vi "Obtain Request Events.vi"(8 "error in":errorcluster, 10 "Create New? (F)":bool) -> (0 "error out":errorcluster, 2 "USB IO Request Events":T1)   [LabVIEW 2025, in "USB IO.lvlib"]
doc: "This VI Obtains/Creates the Requests events that will be used for other modules to communicate with the module that owns this VI. These Requests events will be accessed only via Public API methods for this module.\n\n<b>NOTE</b>: The contents of this VI are automatically generated and modified by the <b>Tools > DQMH Consortium > DQMH</b> utilities. Consider using those utilities instead of making your own modifications to this VI.\n_____\nBased on DQMH Dev Tools: Project Template 7.1.2.1547."
uses:
  USB IO.lvlib
  Request Events--cluster.ctl
  Stop Argument--cluster.ctl
  Show Panel Argument--cluster.ctl
  Hide Panel Argument--cluster.ctl
  Show Diagram Argument--cluster.ctl
  Get Module Execution Status Argument--cluster.ctl
  Display Lines Argument--cluster.ctl
  Display Lines (Reply Payload)--cluster.ctl
  select child Argument--cluster.ctl
  Classes/Hardware Selection.ctl
  select child (Reply Payload)--cluster.ctl
  read config Argument--cluster.ctl
  read config (Reply Payload)--cluster.ctl
  init Argument--cluster.ctl
  init (Reply Payload)--cluster.ctl
  init device Argument--cluster.ctl
  init device (Reply Payload)--cluster.ctl
  stop device Argument--cluster.ctl
  stop device (Reply Payload)--cluster.ctl
  analog read Argument--cluster.ctl
  analog read (Reply Payload)--cluster.ctl
  Controls/Numeric Voltage.ctl
  digital write Argument--cluster.ctl
  digital write (Reply Payload)--cluster.ctl
panel:
  # "NOTE: The contents of this VI are automatically generated and modified by the Tools > DQMH Consortium > DQMH utilities. Consider using those utilities instead of making your own modifications to this VI."
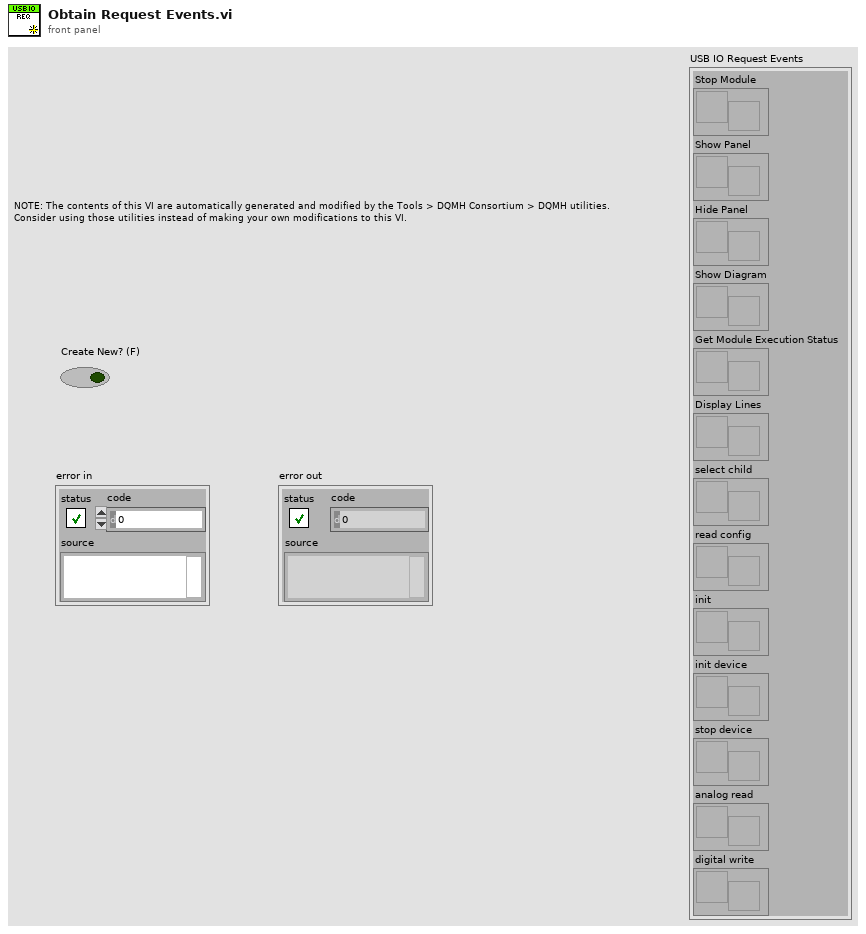
[diagram p1: front panel]
types:
  T1 = typedef "USB IO.lvlib/Request Events--cluster.ctl" = cluster{"Stop Module":refnum<user-event>, "Show Panel":refnum<user-event>, "Hide Panel":refnum<user-event>, "Show Diagram":refnum<user-event>, "Get Module Execution Status":refnum<user-event>, "Display Lines":refnum<user-event>, "select child":refnum<user-event>, "read config":refnum<user-event>, "init":refnum<user-event>, "init device":refnum<user-event>, "stop device":refnum<user-event>, "analog read":refnum<user-event>, "digital write":refnum<user-event>}
  T2 = typedef "USB IO.lvlib/digital write Argument--cluster.ctl" = cluster{"Module ID":i32, "Line":string, "On/Off":bool, "Wait Notifier":refnum<notifier>, "wait for reply":bool}
  T3 = typedef "USB IO.lvlib/analog read Argument--cluster.ctl" = cluster{"Module ID":i32, "Line":string, "Wait Notifier":refnum<notifier>, "wait for reply":bool}
  T4 = typedef "USB IO.lvlib/stop device Argument--cluster.ctl" = cluster{"Module ID":i32, "Wait Notifier":refnum<notifier>, "wait for reply":bool}
  T5 = typedef "USB IO.lvlib/init device Argument--cluster.ctl" = cluster{"Module ID":i32, "Variant":variant, "Wait Notifier":refnum<notifier>, "wait for reply":bool}
  T6 = typedef "USB IO.lvlib/init Argument--cluster.ctl" = cluster{"Module ID":i32, "Wait Notifier":refnum<notifier>, "wait for reply":bool}
  T7 = typedef "USB IO.lvlib/read config Argument--cluster.ctl" = cluster{"Module ID":i32, "Path":path, "Wait Notifier":refnum<notifier>, "wait for reply":bool}
  T8 = typedef "USB IO.lvlib/select child Argument--cluster.ctl" = cluster{"Module ID":i32, "Hardware":T9, "Wait Notifier":refnum<notifier>, "wait for reply":bool}
  T9 = typedef "Hardware Selection.ctl" = enum16{"Simulation", "USB-6000", "USB-6001", "Arduino Uno"}
  T10 = typedef "USB IO.lvlib/Display Lines Argument--cluster.ctl" = cluster{"Module ID":i32, "Wait Notifier":refnum<notifier>, "wait for reply":bool}
  T11 = typedef "USB IO.lvlib/Get Module Execution Status Argument--cluster.ctl" = cluster{"Module ID":i32, "Running?":bool}
  T12 = typedef "USB IO.lvlib/Show Diagram Argument--cluster.ctl" = cluster{"Module ID":i32, "Debug?":bool}
  T13 = typedef "USB IO.lvlib/Show Panel Argument--cluster.ctl" = cluster{"Module ID":i32, "Show Panel?":bool}
  T14 = typedef "USB IO.lvlib/Hide Panel Argument--cluster.ctl" = cluster{"Module ID":i32, "Hide Panel?":bool}
  T15 = typedef "USB IO.lvlib/Stop Argument--cluster.ctl" = cluster{"Module ID":i32, "Origin":string, "Exit via Stop Module Req?":bool, "Wait for Module to stop?":bool}
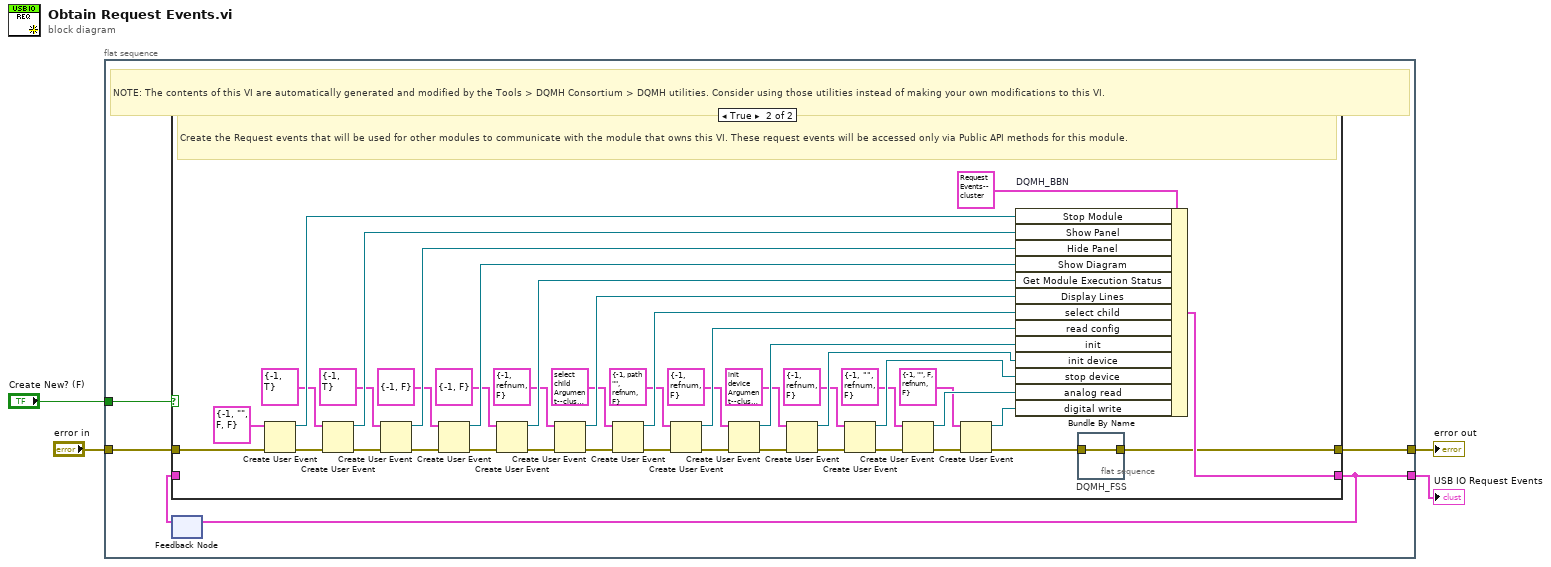
[diagram p0: block diagram]
diagram:
  n1 = flat-sequence {
    tunnel: [w9] -> w4
    tunnel: "error in" -> [w8]
    tunnel: [w6] -> w2
    tunnel: "Create New? (F)" -> [w5]
    frame #0 {
      # "NOTE: The contents of this VI are automatically generated and modified by the Tools > DQMH Consortium > DQMH utilities. Consider using those utilities instead of making your own modifications to this VI."
      n2 = feedback #1() -> (w7:T1)  [unwired: 1 in]
      n3 = case shown="True" w5 {
        tunnel: [w10 w42] -> w9
        tunnel: w8 -> [w10 w54]
        tunnel: [w11 w51] -> w6
        tunnel: w7 -> [w11 _]
        frame False {
        }
        frame True {
          # "Create the Request events that will be used for other modules to communicate with the module that owns this VI. These request events will be accessed only via Public API methods for this module."
          n4 = Create User Event(user event datatype=T15 {"Module ID"=-1, "Origin"="", "Exit via Stop Module Req?"=FALSE, "Wait for Module to stop?"=FALSE} ("Stop Argument"), error in=w54) -> (user event=w52:refnum<user-event>, error out=w49:errorcluster)
          n5 = Create User Event(user event datatype=T13 {"Module ID"=-1, "Show Panel?"=TRUE} ("Show Panel Argument"), error in=w49) -> (user event=w48:refnum<user-event>, error out=w46:errorcluster)
          n6 = Create User Event(user event datatype=T14 {"Module ID"=-1, "Hide Panel?"=TRUE} ("Hide Panel"), error in=w46) -> (user event=w45:refnum<user-event>, error out=w44:errorcluster)
          n7 = Create User Event(user event datatype=T12 {"Module ID"=-1, "Debug?"=FALSE} ("Show Diagram Argument"), error in=w44) -> (user event=w40:refnum<user-event>, error out=w41:errorcluster)
          n8 = Create User Event(user event datatype=T11 {"Module ID"=-1, "Running?"=FALSE} ("Get Module Execution Status Argument"), error in=w41) -> (user event=w37:refnum<user-event>, error out=w38:errorcluster)
          n9 = Create User Event(user event datatype=T10 {"Module ID"=-1, "Wait Notifier"=refnum, "wait for reply"=FALSE} ("Display Lines Argument"), error in=w38) -> (user event=w34:refnum<user-event>, error out=w35:errorcluster)
          n10 = Create User Event(user event datatype=T8 {"Module ID"=-1, "Hardware"=enum."USB-6000", "Wait Notifier"=refnum, "wait for reply"=FALSE} ("select child Argument"), error in=w35) -> (user event=w31:refnum<user-event>, error out=w32:errorcluster)
          n11 = Create User Event(user event datatype=T7 {"Module ID"=-1, "Path"=path "", "Wait Notifier"=refnum, "wait for reply"=FALSE} ("read config Argument"), error in=w32) -> (user event=w28:refnum<user-event>, error out=w29:errorcluster)
          n12 = Create User Event(user event datatype=T6 {"Module ID"=-1, "Wait Notifier"=refnum, "wait for reply"=FALSE} ("init Argument"), error in=w29) -> (user event=w25:refnum<user-event>, error out=w26:errorcluster)
          n13 = Create User Event(user event datatype=T5 {"Module ID"=-1, "Variant"=variant, "Wait Notifier"=refnum, "wait for reply"=FALSE} ("init device Argument"), error in=w26) -> (user event=w22:refnum<user-event>, error out=w23:errorcluster)
          n14 = Create User Event(user event datatype=T4 {"Module ID"=-1, "Wait Notifier"=refnum, "wait for reply"=FALSE} ("stop device Argument"), error in=w23) -> (user event=w19:refnum<user-event>, error out=w20:errorcluster)
          n15 = Create User Event(user event datatype=T3 {"Module ID"=-1, "Line"="", "Wait Notifier"=refnum, "wait for reply"=FALSE} ("analog read Argument"), error in=w20) -> (user event=w16:refnum<user-event>, error out=w17:errorcluster)
          n16 = Create User Event(user event datatype=T2 {"Module ID"=-1, "Line"="", "On/Off"=FALSE, "Wait Notifier"=refnum, "wait for reply"=FALSE} ("digital write Argument"), error in=w17) -> (user event=w13:refnum<user-event>, error out=w14:errorcluster)
          n17 = Bundle By Name "DQMH_BBN"(cluster=T1 {"Stop Module"=refnum, "Show Panel"=refnum, "Hide Panel"=refnum, "Show Diagram"=refnum, "Get Module Execution Status"=refnum, "Display Lines"=refnum, "select child"=refnum, "read config"=refnum, "init"=refnum, "init device"=refnum, "stop device"=refnum, "analog read"=refnum, "digital write"=refnum} ("output cluster"), "Stop Module"=w52, "Show Panel"=w48, "Hide Panel"=w45, "Show Diagram"=w40, "Get Module Execution Status"=w37, "Display Lines"=w34, "select child"=w31, "read config"=w28, "init"=w25, "init device"=w22, "stop device"=w19, "analog read"=w16, "digital write"=w13) -> (w51:T1)
          n18 = flat-sequence "DQMH_FSS" {
            tunnel: w14 -> [w55]
            tunnel: [w55] -> w42
            frame #0 {
            }
          }
        }
      }
      n19 = feedback-in #1(w6) -> ()
    }
  }
  "USB IO Request Events" <- w2
  "error out" <- w4
